vi "fgv_stop-point_delay.vi"(7 "cmd":enum16{"init", "read", "write"}(ring), 8 "error in":errorcluster, 11 "dt":dbl) -> (0 "error out":errorcluster, 3 "stop dt out":dbl)   [LabVIEW 2019]
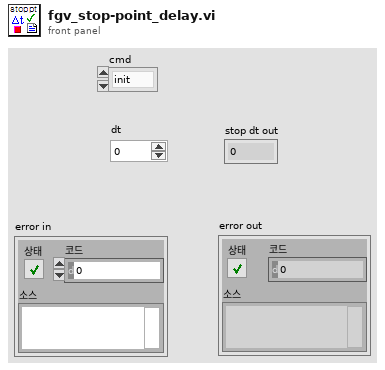
[diagram p1: front panel]
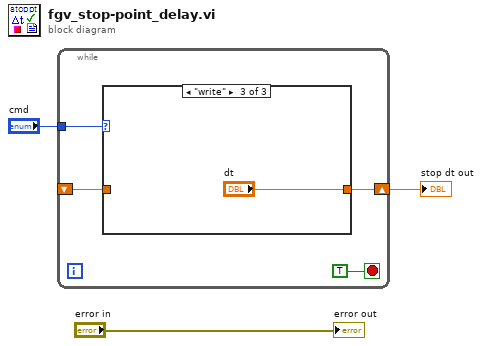
[diagram p0: block diagram]
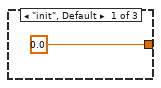
[diagram p2: hidden frame]
diagram:
  n1 = while {
    tunnel: "cmd" -> [w6]
    shift-right: [w5] -> w1
    shift-left: _ -> [w4]
    stop <- TRUE stop-if-true
    n2 = case shown="\"write\"" w6 {
      tunnel: [0.0 ("dt") w9 "dt"] -> w5
      tunnel: w4 -> [_ w9 _]
      frame "init", Default {
      }
      frame "read" {
      }
      frame "write" {
      }
    }
  }
  "stop dt out" <- w1
  "error out" <- "error in"
